vi "Assert Not Refnum.vi"(7 "Message (\"\")":string, 8 "error in (no error)":errorcluster, 10 "Refnum":variant) -> (0 "error out":errorcluster)   [LabVIEW 2017, in "Transparent Assertions.lvlib"]
doc: "Asserts that a refnum is not valid. Returns an error if the assertion fails, and optionally appends a custom message to the error."
uses:
  Transparent Assertions.lvlib
  LogicalNot/LogicalNot.lvclass
  IsRefnum/IsRefnum.lvclass
  C:/Users/pasca/Projects/Home/TransparentAssertions/src/Transparent Assertions/Constraints/Constraint/Constraint.lvclass
  UnaryOperator/UnaryOperator.lvclass
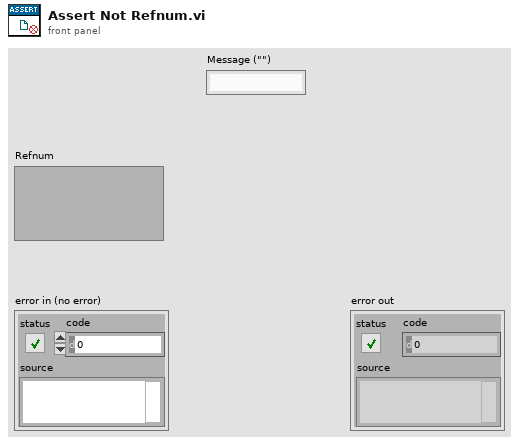
[diagram p1: front panel]
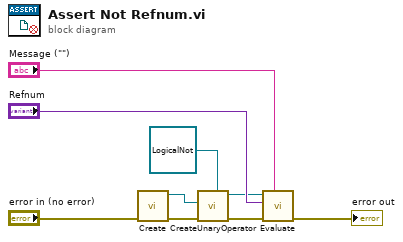
[diagram p0: block diagram]
diagram:
  n1 = call "Create.vi"("error in (no error)"="error in (no error)") -> ("error out"=w8:errorcluster, "IsRefnum"=w4:refnum<class "IsRefnum.lvclass">)  [unwired: 9 in]
  n2 = call-dynamic "CreateUnaryOperator.vi"("UnaryOperator In"=refnum<class "LogicalNot.lvclass"> refnum, "error in (no error)"=w8, "Constraint"=w4) -> ("error out"=w5:errorcluster, "UnaryOperator"=w2:refnum<class "UnaryOperator.lvclass">)  [unwired: 7 in]
  n3 = call-dynamic "Evaluate.vi"("Message (\"\")"="Message (\"\")", "error in (no error)"=w5, "Actual"="Refnum", "Constraint in"=w2) -> ("error out"=→"error out":errorcluster)  [unwired: 6 in, 1 out]
